vi "Generate Waveform.vi"(0 "signal configuration":refnum<class "SV Square.lvclass">, 5 "template waveform":waveform(dbl), 9 "samples":i32, 11 "error in (no error)":errorcluster) -> (4 "signal configuration":refnum<class "SV Square.lvclass">, 6 "square waveform":waveform(dbl), 10 "samples":i32, 15 "error out":errorcluster)   [LabVIEW 2017, in "SV Square.lvclass"]
uses:
  <vilib>/addons/_NISVFA/_Generation/Signal Generation/SV Square/SV Square.lvclass
  C:/Program Files (x86)/National Instruments/LabVIEW 2017/vi.lib/addons/_NISVFA/_Generation/Signal Generation/SV Signal/SV Signal.lvclass
  C:/Program Files (x86)/National Instruments/LabVIEW 2017/vi.lib/addons/_NISVFA/_Generation/Signal Generation/SV Function/SV Function.lvclass
  <vilib>/addons/_NISVFA/_Generation/Signal Generation/SV Signal/sv_Signal State Attribute.ctl
  <vilib>/addons/_NISVFA/_Generation/Signal Generation/SV Square/SV Square.lvclass/SV Square.ctl
  <vilib>/addons/_NISVFA/_Generation/Signal Generation/SV Signal/Read Sample Rate.vi
  <vilib>/Analysis/NI_AALBase.lvlib
  <vilib>/addons/_NISVFA/_Generation/Signal Generation/SV Function/SV Function.lvclass
  <vilib>/addons/_NISVFA/_Generation/Signal Generation/SV Signal/SV Signal.lvclass
  <vilib>/measure/NI_MABase.lvlib
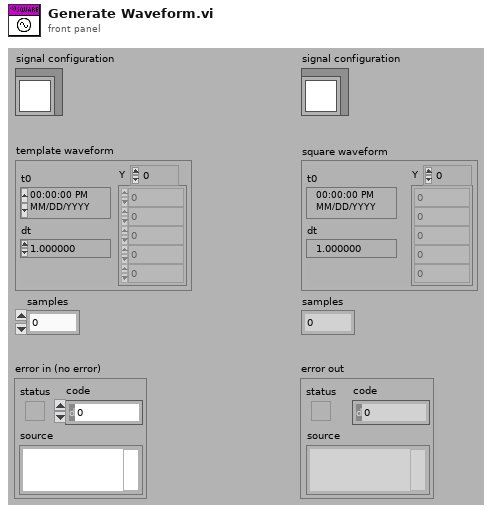
[diagram p1: front panel]
types:
  T1 = typedef "SV Signal.lvclass/sv_Signal State Attribute.ctl" = string
  T2 = typedef "SV Signal.lvclass/sv_System Timing Model.ctl" = i64
  T3 = typedef "SV Signal.lvclass/sv_Generation State.ctl" = enum16{"Idle", "Ramp Up", "Pre-Measurement Settling", "Measurement", "Post-Measurement Settling", "Discrete Sweep Transition", "Ramp Down", "Update"}
  T4 = cluster{"system timing model":T2, "state":cluster{"RESET":bool, "generator timestamp":timestamp, "elapsed seconds":dbl, "elapsed samples":u64, "generation state":T3, "time offset at state":dbl, "samples generated at state":u64, "signal state":variant}, "duration of state":dbl, "samples remaining at state":i32}
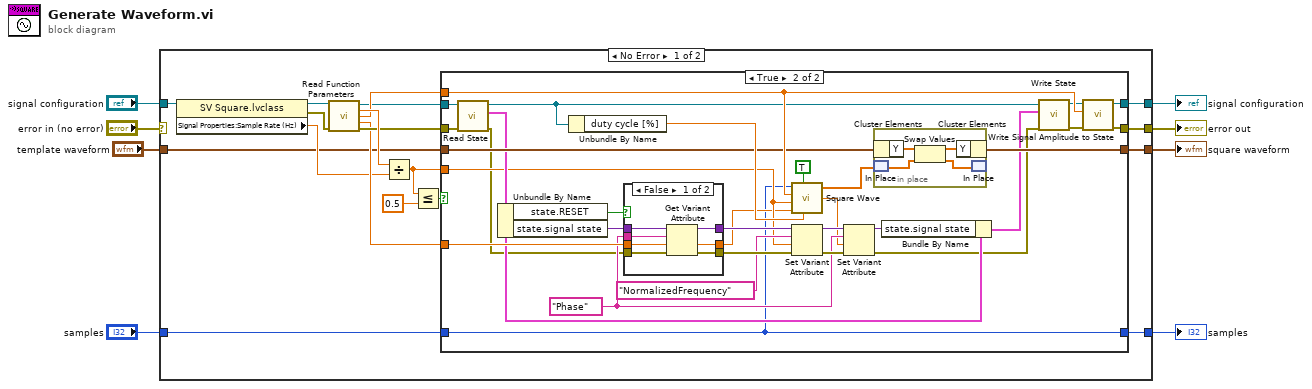
[diagram p0: block diagram]
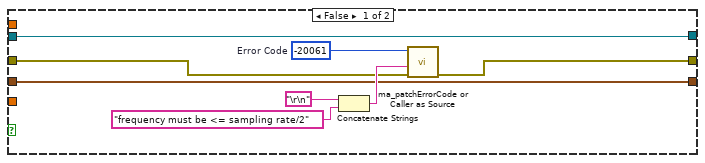
[diagram p2: hidden frame]
diagram:
  n1 = case shown="No Error" "error in (no error)" {
    selector: "error in (no error)" -> [_ w81]
    tunnel: [w15 w81] -> w7
    tunnel: [w16 w80] -> w5
    tunnel: "signal configuration" -> [w14 w80]
    tunnel: [w19 _] -> w4
    tunnel: [w9 _] -> w3
    tunnel: "samples" -> [w17 _]
    tunnel: "template waveform" -> [w18 _]
    frame No Error {
      n2 = property class="SV Square.lvclass"(reference=w14) -> (reference out=w23:refnum<class "SV Square.lvclass">, error out=w22:errorcluster, "Signal Properties:Sample Rate (Hz)"=w21:dbl)  [unwired: 1 in]
      n3 = call <vilib>:"Read Function Parameters.vi"("signal configuration"=w23, "error in (no error)"=w22) -> ("signal configuration"=w13:refnum<class "SV Square.lvclass">, "frequency_Hz"=w26:dbl, "amplitude"=w20:dbl, "initial_phase_deg"=w24:dbl, "error out"=w25:errorcluster)  [unwired: 8 in, 1 out]
      n4 = Divide(x=w26, y=w21) -> (x/y=w11:dbl)
      n5 = Less Or Equal?(x=w11, y=0.5) -> (x <= y?=w10:bool)
      n6 = case shown="True" w10 {
        tunnel: w25 -> [w29 w41]
        tunnel: w24 -> [_ w65]
        tunnel: w20 -> [_ w64]
        tunnel: [w27 w61] -> w19
        tunnel: w18 -> [w27 w59]
        tunnel: w17 -> [_ w42]
        tunnel: w11 -> [_ w49]
        tunnel: [w30 w37] -> w16
        tunnel: [w28 w36] -> w15
        tunnel: w13 -> [w30 w43]
        tunnel: [_ w42] -> w9
        frame False {
          w31 = -20061  # Error Code
          n7 = Concatenate Strings("\r\n", "frequency must be <= sampling rate/2" ("freq error message")) -> (w34:string)
          n8 = call <vilib>:"ma_patchErrorCode or Caller as Source.vi"("error in (no error)"=w29, "string to append to source"=w34, "error code"=w31) -> ("error out"=w28:errorcluster)  [unwired: 8 in]
        }
        frame True {
          w50 = T1 "Phase" ("name")
          n9 = call <vilib>:"Read State.vi"("error in (no error)"=w41, "signal configuration"=w43) -> ("error out"=w40:errorcluster, "generator state"=w54:T4, "signal configuration"=w39:refnum<class "SV Square.lvclass">)  [unwired: 7 in]
          n10 = Unbundle By Name(w54) -> ("state.RESET"=w35:bool, "state.signal state"=w55:variant)
          n11 = Unbundle By Name(w39) -> ("duty cycle [%]"=w60:dbl)
          n12 = case shown="False" w35 {
            tunnel: w55 -> [w72 w74]
            tunnel: w65 -> [w71 w75]
            tunnel: [w70 w75] -> w47
            tunnel: [w69 w74] -> w56
            tunnel: w40 -> [w68 w73]
            tunnel: [w67 w73] -> w58
            tunnel: w50 -> [w66 _]
            frame False {
              n13 = Get Variant Attribute(Variant=w72, name=w66, default value (empty Variant)=w71, error in=w68) -> (duplicate Variant=w69:variant, value=w70:dbl, error out=w67:errorcluster)  [unwired: 1 out]
            }
            frame True {
            }
          }
          n14 = call <vilib>:"Square Wave.vi"("samples"=w42, "reset phase"=TRUE, "amplitude"=w64, "frequency"=w49, "duty cycle (%)"=w60, "phase in"=w47) -> ("square wave"=w63:dbl[], "phase out"=w48:dbl)  [unwired: 1 out]
          n15 = Set Variant Attribute(Variant=w56, name=T1 "NormalizedFrequency", value=w49, error in=w58) -> (Variant out=w53:variant, error out=w51:errorcluster)  [unwired: 1 out]
          n16 = Set Variant Attribute(Variant=w53, name=w50, value=w48, error in=w51) -> (Variant out=w52:variant, error out=w38:errorcluster)  [unwired: 1 out]
          n17 = in-place {
            n18 = in-place-cluster #1(w59) -> ("Y"=w79:dbl[])
            n19 = in-place-match #2(w63) -> (w77:dbl[])
            n20 = Swap Values(12:w79, 14:w77) -> (1:w78:dbl[], 3:w76:dbl[])  [unwired: 1 in]
            n21 = in-place-cluster #1("Y"=w78) -> (w61:waveform(dbl))
            n22 = in-place-match #2(w76) -> ()  [unwired: 1 out]
          }
          n23 = Bundle By Name(cluster=w54, "state.signal state"=w52) -> (w46:T4)
          n24 = call <vilib>:"Write State.vi"("error in (no error)"=w38, "generator state"=w46, "signal configuration"=w39) -> ("error out"=w44:errorcluster, "signal configuration"=w45:refnum<class "SV Square.lvclass">)  [unwired: 7 in]
          n25 = call <vilib>:"Write Signal Amplitude to State.vi"("error in (no error)"=w44, "amplitude"=w64, "SV Signal in"=w45) -> ("error out"=w36:errorcluster, "SV Signal out"=w37:refnum<class "SV Square.lvclass">)  [unwired: 7 in]
        }
      }
    }
    frame Error {
    }
  }
  "error out" <- w7
  "signal configuration" <- w5
  "square waveform" <- w4
  "samples" <- w3
